vi "Mutate.LVInstaller.vi"   [LabVIEW 2013, in "VeriStand Steps Version Mutation.lvlib"]
uses:
  VeriStand Steps Version Mutation.lvlib
types:
  T1 = typedef "VeriStand Steps Version Mutation.lvlib/LVInstallerMutationSession.ctl" = cluster{"Installer Build Specification Ref":refnum<vi>, "Project reference out":refnum<vi>, "Installer Project Path":path}
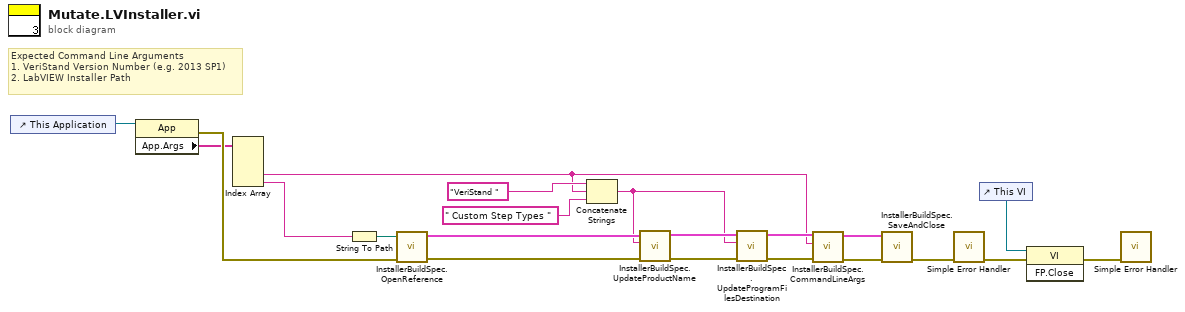
[diagram p0: block diagram]
diagram:
  # "Expected Command Line Arguments\n1. VeriStand Version Number (e.g. 2013 SP1)\n2. LabVIEW Installer Path"
  n1 = control-ref of="This Application"() -> (w13:refnum<vi>)
  n2 = property class="App"(reference=w13) -> (error out=w12:errorcluster, "App.Args"=w8:string[])  [unwired: 1 in, 1 out]
  n3 = Index Array(array=w8) -> (element #3=w6:string, element #4=w5:string)  [unwired: 4 in, 2 out]
  n4 = String To Path(string=w5) -> (path=w7:path)
  n5 = call "InstallerBuildSpec.OpenReference.vi"("error in (no error)"=w12, "Installer Project Path"=w7) -> ("error out"=w21:errorcluster, "InstallerSession"=w20:T1)  [unwired: 8 in]
  n6 = Concatenate Strings("VeriStand " ("string"), w6, " Custom Step Types " ("string")) -> (w9:string)
  n7 = call "InstallerBuildSpec.UpdateProductName.vi"("error in (no error)"=w21, "Installer Product Name"=w9, "InstallerMutationSession"=w20) -> ("error out"=w19:errorcluster, "InstallerMutationSession out"=w18:T1)  [unwired: 7 in]
  n8 = call "InstallerBuildSpec.UpdateProgramFilesDestination.vi"("error in (no error)"=w19, "New Application Directory Name"=w9, "InstallerMutationSession"=w18) -> ("error out"=w16:errorcluster, "InstallerMutationSession out"=w17:T1)  [unwired: 7 in]
  n9 = call "InstallerBuildSpec.CommandLineArgs.vi"("error in (no error)"=w16, "New Version Command Line Argument"=w6, "InstallerMutationSession"=w17) -> ("error out"=w14:errorcluster, "InstallerMutationSession out"=w15:T1)  [unwired: 7 in]
  n10 = call "InstallerBuildSpec.SaveAndClose.vi"("error in (no error)"=w14, "InstallerMutationSession"=w15) -> ("error out"=w4:errorcluster)  [unwired: 9 in]
  n11 = call <vilib>:"Simple Error Handler.vi"("error in (no error)"=w4) -> ("error out"=w3:errorcluster)  [unwired: 4 in, 4 out]
  n12 = control-ref of="This VI"() -> (w2:refnum<vi>)
  n13 = invoke class="VI" method="FP.Close"(reference=w2, error in=w3) -> (error out=w1:errorcluster)  [unwired: 1 in, 2 out]
  n14 = call <vilib>:"Simple Error Handler.vi"("error in (no error)"=w1) -> ()  [unwired: 4 in, 5 out]
